vi "Autonomous Independent.vi"() -> ()   [LabVIEW 2017]
doc: "This VI is called when autonomous begins, and will automatically be terminated when autonomous ends. You can carry out timed or sensor driven robot movement independently without needing to return to the caller."
uses:
  <vilib>/Rock Robotics/WPI/DriverStation/WPI_DriverStationAllianceInfo.ctl
  <vilib>/Rock Robotics/WPI/Utilities/WPI_GetSetVariantRefNum.vi
  <vilib>/Rock Robotics/Network Tables/NT Read String.vi
  <vilib>/Rock Robotics/Network Tables/NT Write Numeric Array.vi
  <vilib>/Rock Robotics/WPI/RobotDrive/WPI_RobotDriveArcadeDrive_Standard(NoSaturation).vi
panel:
  in  "Test Recording":T1
  in  "Wrist Backward Delivery Recording":cluster{dbl, u32}[](array[cluster])
  in  "Shoulder Backward Delivery Recording":cluster{dbl, u32}[](array[cluster])
  in  "Wrist Delivery Recording":cluster{dbl, u32}[](array[cluster])
  in  "Shoulder Delivery Recording":cluster{dbl, u32}[](array[cluster])
  in  "Switch to Far Scale":T1
  in  "Switch to Close Scale":T1
  in  "Wrist Switch Delivery Recording":cluster{dbl, u32}[](array[cluster])
  in  "Start to Switch":T1
  out "Current Movement, for debugging":T2 {"Y Joystick Value" scale=1.0..-1.0; "X Joystick Value" scale=-1.0..1.0}
  in  "Array of robot movements":T3(array[cluster])=[{"X Joystick Value"=0.39393939393939403, "Y Joystick Value"=0.0, "Delay (sec)"=1.0, "Movement Name"="turn"}, {"X Joystick Value"=-0.3737373737373737, "Y Joystick Value"=0.0, "Delay (sec)"=1.0, "Movement Name"="turn back"}] {"Y Joystick Value" scale=1.0..-1.0; "X Joystick Value" scale=-1.0..1.0}
  # "Todo:\n-Invert the axis\n-Arm recordings\n-Floor Recordings\n-PID Values for Arms\n-PID Values for Floor"
  # "Be sure to right-click and choose Data Operations>>Make Current Value default if you want to save the array values with the VI"
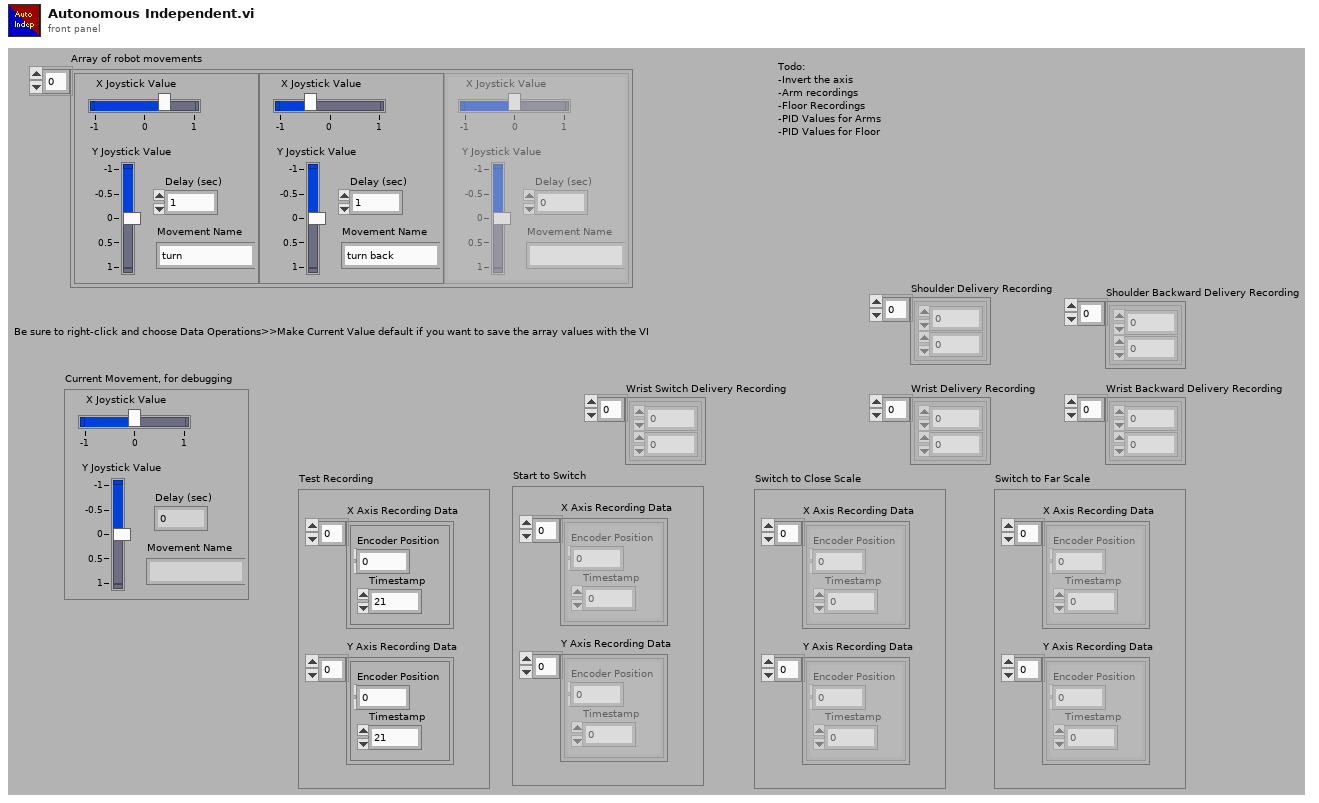
[diagram p1: front panel]
types:
  T1 = cluster{"X Axis Recording Data":cluster{"Encoder Position":dbl, "Timestamp":i32}[], "Y Axis Recording Data":cluster{"Encoder Position":dbl, "Timestamp":i32}[]}
  T2 = cluster{"X Joystick Value":dbl, "Y Joystick Value":dbl, "Delay (sec)":dbl, "Movement Name":string}
  T3 = cluster{"X Joystick Value":dbl, "Y Joystick Value":dbl, "Delay (sec)":dbl, "Movement Name":string}[]
  T4 = typedef "WPI_DriverStationAllianceInfo.ctl" = enum16{"Red", "Blue", "Invalid"}
  T5 = typedef "WPI_JoystickDevRef.ctl" = cluster{"Device":T6}
  T6 = typedef "WPI_JoystickDeviceEnum.ctl" = enum16{"USB 0", "USB 1", "USB 2", "USB 3", "USB 4", "USB 5"}
  T7 = typedef "WPI_RobotDriveDevRef.ctl" = cluster{"DevStatus":errorcluster, "Motors[]":T8[], "Square Inputs":bool, "Max Output":dbl}
  T8 = typedef "WPI_MotorControlDeviceRef.ctl" = cluster{"DeviceStatus":errorcluster, "Type":T9, "PWM":cluster{"PWM Channel":T10, "DeadBand":T11}, "CAN":cluster{"Device Number":u8, "SetOutput VI Ref":variant, "GetOutput VI Ref":variant, "Enable VI Ref":variant, "Disable VI Ref":variant, "Data":variant}, "Invert":bool, "DIO PWM":cluster{"PWM \"Enable\" Channel":T10, "DIOChannel":T12, "PWM Rate":dbl}}
  T9 = typedef "WPI_MotorControlType.ctl" = enum16{"PWM", "CAN", "DIO PWM"}
  T10 = typedef "FPGA_DIOPWMChannel.ctl" = enum8{"PWM 0", "PWM 1", "PWM 2", "PWM 3", "PWM 4", "PWM 5", "PWM 6", "PWM 7", "PWM 8", "PWM 9", "PWM MXP 0", "PWM MXP 1", "PWM MXP 2", "PWM MXP 3", "PWM MXP 4", "PWM MXP 5", "PWM MXP 6", "PWM MXP 7", "PWM MXP 8", "PWM MXP 9", "Invalid"}
  T11 = typedef "WPI_PWMDeadband.ctl" = cluster{"Name":string, "maxPositivePwm":i32, "minPositivePwm":i32, "centerPwm":i32, "maxNegativePwm":i32, "minNegativePwm":i32, "angularRange":u16}
  T12 = typedef "FPGA_DIOChannel.ctl" = enum8{"DIO 0", "DIO 1", "DIO 2", "DIO 3", "DIO 4", "DIO 5", "DIO 6", "DIO 7", "DIO 8", "DIO 9", "DIO MXP 0", "DIO MXP 1", "DIO MXP 2", "DIO MXP 3", "DIO MXP 4", "DIO MXP 5", "DIO MXP 6", "DIO MXP 7", "DIO MXP 8", "DIO MXP 9", "DIO MXP 10", "DIO MXP 11", "DIO MXP 12", "DIO MXP 13", "DIO MXP 14", "DIO MXP 15", "SPI Port CS1", "SPI Port CS2", "SPI Port CS3", "SPI Port MISO", "SPI Port MOSI", "Invalid"}
  T13 = typedef "WPI_EncoderDevRef.ctl" = cluster{"DevStatus":errorcluster, "EncoderIndex":T14, "CounterIndex":T15, "DistancePerCount":dbl, "Decoding Type":T16}
  T14 = typedef "FPGA_EncoderIdx.ctl" = enum8{"Enc 0", "Enc 1", "Enc 2", "Enc 3", "Enc 4", "Enc 5", "Enc 6", "Enc 7", "Invalid"}
  T15 = typedef "FPGA_CounterCtrSystemIndex.ctl" = enum8{"Ctr 0", "Ctr 1", "Ctr 2", "Ctr 3", "Ctr 4", "Ctr 5", "Ctr 6", "Ctr 7", "Invalid"}
  T16 = typedef "WPI_EncoderType.ctl" = enum16{"1x", "2x", "4x"}
  T17 = cluster{"refnum name":string, "EncoderDevRef":T13}
  T18 = cluster{"MotorControlDevRef":T8, "MotorControlDevRef":T8}
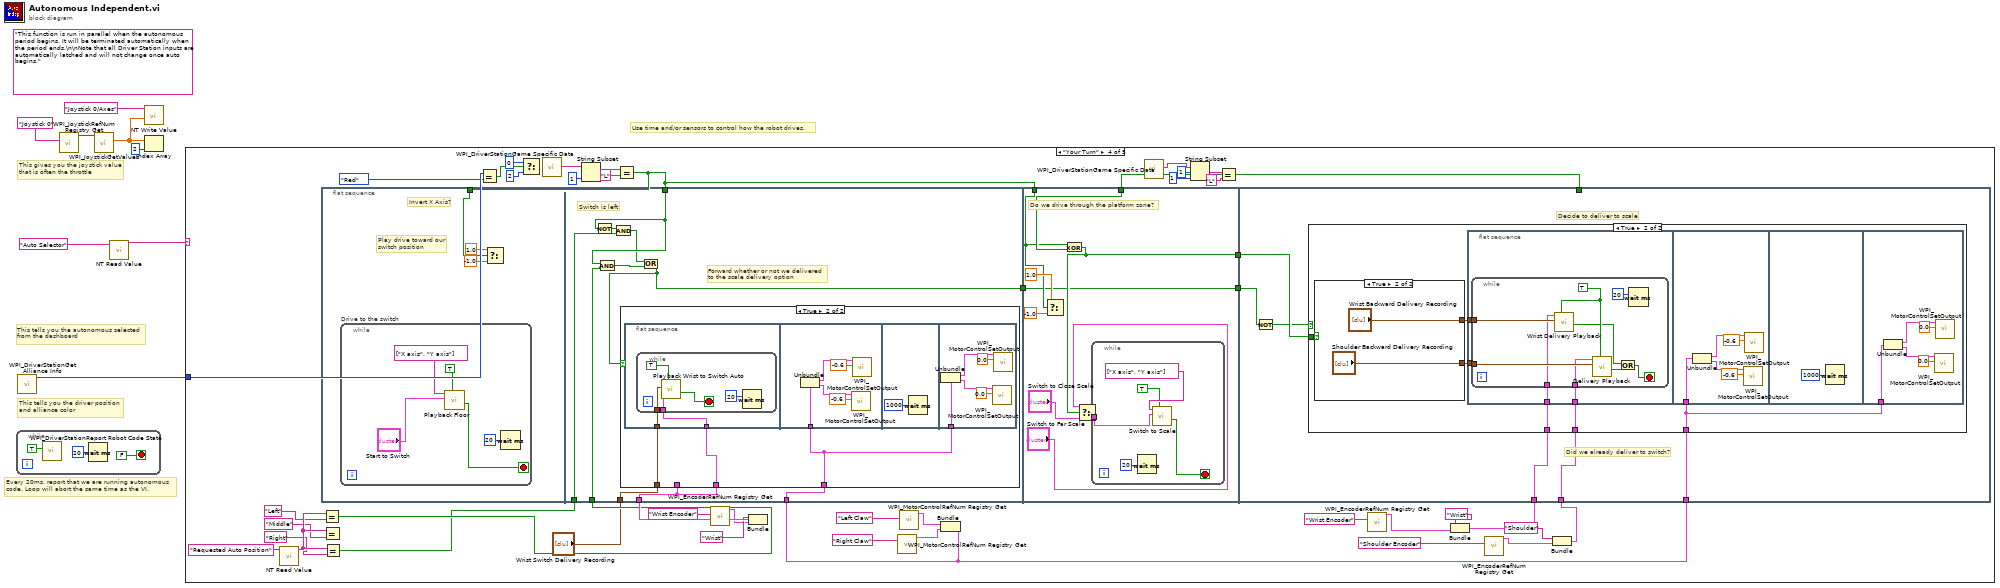
[diagram p0: block diagram]
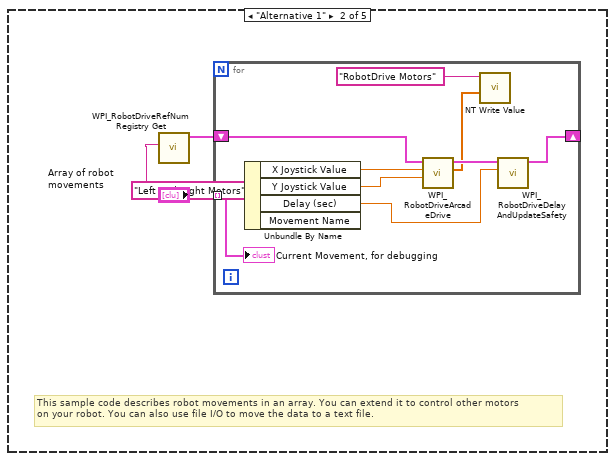
[diagram p3: hidden frame]
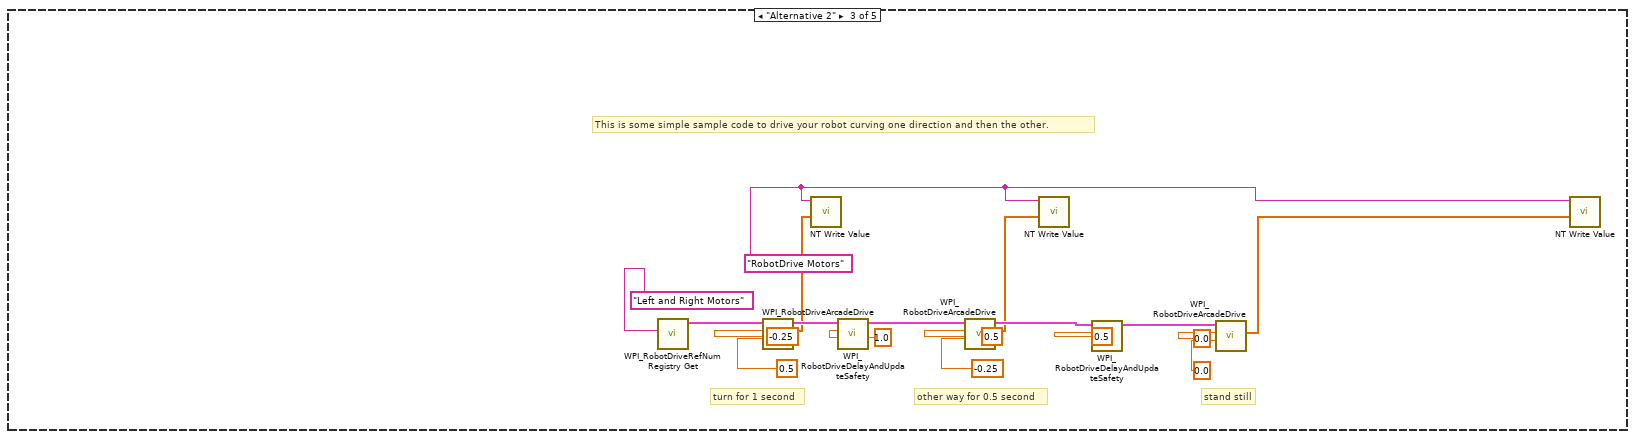
[diagram p4: hidden frame]
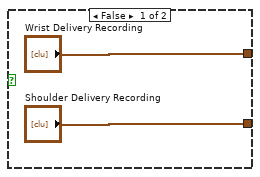
[diagram p7: hidden frame]
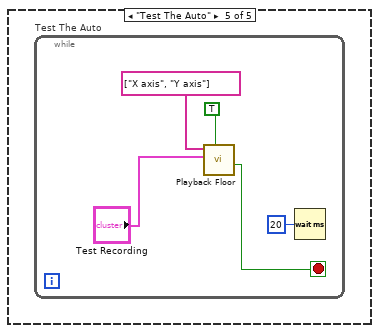
[diagram p8: hidden frame]
diagram:
  (unwired) "This function is run in parallel when the autonomous period begins. It will be terminated automatically when the period ends.\n\nNote that all Driver Station inputs are automatically latched and will not change once auto begins."
  # "This tells you the autonomous selected\nfrom the dashboard"
  # "Every 20ms, report that we are running autonomous\ncode. Loop will abort the same time as the VI."
  # "This gives you the joystick value\nthat is often the throttle"
  # "Use time and/or sensors to control how the robot drives."
  # "This tells you the driver position\nand alliance color"
  n1 = while {
    stop <- FALSE stop-if-true
    n2 = call <vilib>:"WPI_DriverStationReport Robot Code State.vi"("Autonomous"=TRUE) -> ()  [unwired: 10 in, 1 out]
    n3 = Wait (ms)(milliseconds to wait=u32 20) -> ()  [unwired: 1 out]
  }
  n4 = call <vilib>:"WPI_DriverStationGet Alliance Info.vi"() -> ("Alliance"=w1:T4)  [unwired: 11 out]
  n5 = call <vilib>:"WPI_JoystickRefNum Registry Get.vi"("refnum name"="Joystick 0") -> ("JoystickDevRef"=w7:T5)  [unwired: 1 in, 9 out]
  n6 = call <vilib>:"WPI_JoystickGetValues.vi"("JoystickDevRef"=w7) -> ("Axes"=w3:dbl[])  [unwired: 6 in, 4 out]
  n7 = call-poly <vilib>:"NT Read Value.vi"("Name"="Auto Selector") -> ("String"=w4:string)  [unwired: 9 in, 1 out]
  n8 = call-poly <vilib>:"NT Write Value.vi"("Numeric Array"=w3, "Name"="Joystick 0/Axes") -> ()  [unwired: 9 in, 1 out]
  n9 = Index Array(array=w3, index=2) -> ()  [unwired: 1 out]
  n10 = case shown="\"Your Turn\"" w4 {
    tunnel: w1 -> [_ _ _ w79 _]
    frame Default {
      # "You can put your main auto here, or you can right-click on the case and make any\nother frame be the default case."
      # "This is the frame that will execute if no selection is made, or if it is not recognized"
    }
    frame "Alternative 1" {
      # "This sample code describes robot movements in an array. You can extend it to control other motors\non your robot. You can also use file I/O to move the data to a text file."
      n11 = call <vilib>:"WPI_RobotDriveRefNum Registry Get.vi"("refnum name"="Left and Right Motors") -> ("RobotDriveDevRef"=w13:T7)  [unwired: 1 in, 9 out]
      n12 = for {
        shift-right: [w21] -> _
        shift-left: w13 -> [w22]
        tunnel: "Array of robot movements" -> [w17] mode=indexing
        n13 = Unbundle By Name(w17) -> ("X Joystick Value"=w20:dbl, "Y Joystick Value"=w19:dbl, "Delay (sec)"=w18:dbl)  [unwired: 1 out]
        n14 = call-poly <vilib>:"WPI_RobotDriveArcadeDrive.vi"("Y axis value"=w19, "X axis value"=w20, "RobotDriveDevRef"=w22) -> ("Motor Values"=w15:dbl[], "RobotDriveDevRef"=w23:T7)  [unwired: 1 in, 6 out]
        n15 = call-poly <vilib>:"NT Write Value.vi"("Numeric Array"=w15, "Name"="RobotDrive Motors") -> ()  [unwired: 9 in, 1 out]
        n16 = call <vilib>:"WPI_RobotDriveDelayAndUpdateSafety.vi"("Delay (s)"=w18, "RobotDriveDevRef"=w23) -> ("RobotDriveDevRef 2"=w21:T7)  [unwired: 8 in, 1 out]
        "Current Movement, for debugging" <- w17
      }
    }
    frame "Alternative 2" {
      w25 = "RobotDrive Motors" ("Name")
      # "This is some simple sample code to drive your robot curving one direction and then the other."
      # "stand still"
      # "other way for 0.5 second"
      # "turn for 1 second"
      n17 = call <vilib>:"WPI_RobotDriveRefNum Registry Get.vi"("refnum name"="Left and Right Motors") -> ("RobotDriveDevRef"=w41:T7)  [unwired: 1 in, 9 out]
      n18 = call-poly <vilib>:"WPI_RobotDriveArcadeDrive.vi"("Y axis value"=0.5 ("X axis value"), "X axis value"=-0.25, "RobotDriveDevRef"=w41) -> ("Motor Values"=w24:dbl[], "RobotDriveDevRef"=w34:T7)  [unwired: 1 in, 6 out]
      n19 = call-poly <vilib>:"NT Write Value.vi"("Numeric Array"=w24, "Name"=w25) -> ()  [unwired: 9 in, 1 out]
      n20 = call <vilib>:"WPI_RobotDriveDelayAndUpdateSafety.vi"("Delay (s)"=1.0, "RobotDriveDevRef"=w34) -> ("RobotDriveDevRef 2"=w35:T7)  [unwired: 8 in, 1 out]
      n21 = call-poly <vilib>:"WPI_RobotDriveArcadeDrive.vi"("Y axis value"=-0.25 ("X axis value"), "X axis value"=0.5, "RobotDriveDevRef"=w35) -> ("Motor Values"=w26:dbl[], "RobotDriveDevRef"=w36:T7)  [unwired: 1 in, 6 out]
      n22 = call-poly <vilib>:"NT Write Value.vi"("Numeric Array"=w26, "Name"=w25) -> ()  [unwired: 9 in, 1 out]
      n23 = call <vilib>:"WPI_RobotDriveDelayAndUpdateSafety.vi"("Delay (s)"=0.5, "RobotDriveDevRef"=w36) -> ("RobotDriveDevRef 2"=w37:T7)  [unwired: 8 in, 1 out]
      n24 = call-poly <vilib>:"WPI_RobotDriveArcadeDrive.vi"("Y axis value"=0.0 ("X axis value"), "X axis value"=0.0, "RobotDriveDevRef"=w37) -> ("Motor Values"=w27:dbl[])  [unwired: 1 in, 7 out]
      n25 = call-poly <vilib>:"NT Write Value.vi"("Numeric Array"=w27, "Name"=w25) -> ()  [unwired: 9 in, 1 out]
    }
    frame "Your Turn" {
      n26 = call-poly <vilib>:"NT Read Value.vi"("Name"="Requested Auto Position") -> ("String"=w70:string)  [unwired: 9 in, 1 out]
      n27 = flat-sequence {
        tunnel: w54 -> [w86]
        tunnel: w54 -> [w102]
        tunnel: w65 -> [w96]
        tunnel: w62 -> [w103]
        tunnel: w61 -> [w100]
        tunnel: w53 -> [w97]
        tunnel: "Wrist Switch Delivery Recording" -> [w95]
        tunnel: [w94] -> w42
        tunnel: w55 -> [w133]
        tunnel: w54 -> [w130]
        tunnel: [w126] -> w44
        tunnel: [w125] -> w43
        tunnel: w42 -> [w125]
        tunnel: w55 -> [_]
        tunnel: w53 -> [w144]
        tunnel: w50 -> [w143]
        tunnel: w45 -> [w142]
        tunnel: w44 -> [w141]
        tunnel: w43 -> [w139]
        frame #0 {
          # "Invert X Axis?"
          # "Play drive toward our\nswitch position"
          n28 = while "Drive to the switch" {
            stop <- w91 stop-if-true
            n29 = call "Playback Floor.vi"("Encoder Names"=string[] ["X axis", "Y axis"], "Floor Recording Data"="Start to Switch", "Playback"=TRUE) -> ("End of Playback"=w91:bool)  [unwired: 6 in, 1 out]
            n30 = Wait (ms)(milliseconds to wait=u32 20) -> ()  [unwired: 1 out]
          }
          n31 = Select(t=1.0, s=w86, f=-1.0) -> ()  [unwired: 1 out]
        }
        frame #1 {
          # "Forward whether or not we delivered\nto the scale delivery option"
          # "Switch is left"
          n32 = Not(x=w102) -> (.not. x?=w101:bool)
          n33 = And(x=w102, y=w103) -> (x .and. y?=w98:bool)
          n34 = And(x=w101, y=w100) -> (x .and. y?=w99:bool)
          n35 = Or(x=w99, y=w98) -> (x .or. y?=w94:bool)
          n36 = case shown="True" w94 {
            tunnel: w96 -> [_ _]
            tunnel: w97 -> [_ w106]
            tunnel: w96 -> [_ w105]
            tunnel: w95 -> [_ w104]
            frame False {
              # "Do nothing! We're not delivering here!"
            }
            frame True {
              n37 = flat-sequence {
                tunnel: w105 -> [w108]
                tunnel: w104 -> [w107]
                tunnel: w106 -> [w114]
                tunnel: w106 -> [w120]
                frame #0 {
                  n38 = while {
                    tunnel: w108 -> [w113]
                    tunnel: w107 -> [w110]
                    stop <- w112 stop-if-true
                    n39 = call "Playback Wrist to Switch Auto.vi"("Playback"=TRUE, "Encoder Recording Data"=w110, "Hardware In"=w113) -> ("Finished"=w112:bool)  [unwired: 7 in, 1 out]
                    n40 = Wait (ms)(milliseconds to wait=u32 20) -> ()  [unwired: 1 out]
                  }
                }
                frame #1 {
                  n41 = Unbundle(w114) -> ("MotorControlDevRef"=w118:T8, "MotorControlDevRef"=w117:T8)
                  n42 = call <vilib>:"WPI_MotorControlSetOutput.vi"("Output"=-0.6, "MotorControlDevRef"=w117) -> ()  [unwired: 7 in, 3 out]
                  n43 = call <vilib>:"WPI_MotorControlSetOutput.vi"("Output"=-0.6, "MotorControlDevRef"=w118) -> ()  [unwired: 7 in, 3 out]
                }
                frame #2 {
                  n44 = Wait (ms)(milliseconds to wait=u32 1000) -> ()  [unwired: 1 out]
                }
                frame #3 {
                  n45 = Unbundle(w120) -> ("MotorControlDevRef"=w124:T8, "MotorControlDevRef"=w123:T8)
                  n46 = call <vilib>:"WPI_MotorControlSetOutput.vi"("Output"=0.0, "MotorControlDevRef"=w123) -> ()  [unwired: 7 in, 3 out]
                  n47 = call <vilib>:"WPI_MotorControlSetOutput.vi"("Output"=0.0, "MotorControlDevRef"=w124) -> ()  [unwired: 7 in, 3 out]
                }
              }
            }
          }
        }
        frame #2 {
          # "Do we drive through the platform zone?"
          n48 = Select(t=1.0, s=w130, f=-1.0) -> ()  [unwired: 1 out]
          n49 = Exclusive Or(1:w133, 2:w130) -> (0:w126:bool)
          n50 = Select(t="Switch to Far Scale", s=w126, f="Switch to Close Scale") -> (s? t:f=w127:T1)
          n51 = while {
            tunnel: w127 -> [w134]
            stop <- w137 stop-if-true
            n52 = Wait (ms)(milliseconds to wait=u32 20) -> ()  [unwired: 1 out]
            n53 = call "Switch to Scale.vi"("Encoder Names"=string[] ["X axis", "Y axis"], "Floor Recording Data"=w134, "Playback"=TRUE) -> ("End of Playback"=w137:bool)  [unwired: 6 in, 1 out]
          }
        }
        frame #3 {
          # "Did we already deliver to switch?"
          # "Decide to deliver to scale"
          n54 = Not(x=w139) -> (.not. x?=w140:bool)
          n55 = case shown="True" w140 {
            tunnel: w144 -> [_ w150]
            tunnel: w143 -> [_ w147]
            tunnel: w142 -> [_ w146]
            tunnel: w141 -> [_ w145]
            frame False {
              # "We shall deliver nothing! ah ah ah..."
            }
            frame True {
              n56 = case shown="True" w145 {
                tunnel: ["Shoulder Delivery Recording" "Shoulder Backward Delivery Recording"] -> w149
                tunnel: ["Wrist Delivery Recording" "Wrist Backward Delivery Recording"] -> w148
                frame False {
                }
                frame True {
                }
              }
              n57 = flat-sequence {
                tunnel: w149 -> [w158]
                tunnel: w148 -> [w157]
                tunnel: w147 -> [w156]
                tunnel: w146 -> [w155]
                tunnel: w150 -> [w168]
                tunnel: w150 -> [w174]
                frame #0 {
                  n58 = while {
                    tunnel: w158 -> [w166]
                    tunnel: w157 -> [w165]
                    tunnel: w156 -> [w163]
                    tunnel: w155 -> [w162]
                    stop <- w159 stop-if-true
                    w164 = TRUE
                    n59 = call "Wrist Delivery Playback.vi"("Playback"=w164, "Encoder Recording Data"=w165, "Hardware In"=w162) -> ("Playback Finished"=w160:bool)  [unwired: 7 in, 1 out]
                    n60 = call "Delivery Playback.vi"("Playback"=w164, "Encoder Recording Data"=w166, "Hardware In"=w163) -> ("Finish Playback"=w161:bool)  [unwired: 7 in, 1 out]
                    n61 = Or(x=w160, y=w161) -> (x .or. y?=w159:bool)
                    n62 = Wait (ms)(milliseconds to wait=u32 20) -> ()  [unwired: 1 out]
                  }
                }
                frame #1 {
                  n63 = Unbundle(w168) -> ("MotorControlDevRef"=w172:T8, "MotorControlDevRef"=w171:T8)
                  n64 = call <vilib>:"WPI_MotorControlSetOutput.vi"("Output"=-0.6, "MotorControlDevRef"=w171) -> ()  [unwired: 7 in, 3 out]
                  n65 = call <vilib>:"WPI_MotorControlSetOutput.vi"("Output"=-0.6, "MotorControlDevRef"=w172) -> ()  [unwired: 7 in, 3 out]
                }
                frame #2 {
                  n66 = Wait (ms)(milliseconds to wait=u32 1000) -> ()  [unwired: 1 out]
                }
                frame #3 {
                  n67 = Unbundle(w174) -> ("MotorControlDevRef"=w178:T8, "MotorControlDevRef"=w177:T8)
                  n68 = call <vilib>:"WPI_MotorControlSetOutput.vi"("Output"=0.0, "MotorControlDevRef"=w177) -> ()  [unwired: 7 in, 3 out]
                  n69 = call <vilib>:"WPI_MotorControlSetOutput.vi"("Output"=0.0, "MotorControlDevRef"=w178) -> ()  [unwired: 7 in, 3 out]
                }
              }
            }
          }
        }
      }
      n70 = Equal?(x=w70, y="Left") -> (x = y?=w62:bool)
      n71 = Equal?(x=w70, y="Middle") -> ()  [unwired: 1 out]
      n72 = Equal?(x=w70, y="Right") -> (x = y?=w61:bool)
      n73 = Equal?(x=w79, y=WPI_DriverStationAllianceInfo."Red") -> (x = y?=w77:bool)
      n74 = Select(t=0 ("length (rest)"), s=w77, f=2 ("length (rest)")) -> ()  [unwired: 1 out]
      n75 = call <vilib>:"WPI_DriverStationGame Specific Data.vi"() -> ("Game Specific Data"=w85:string)  [unwired: 11 in]
      n76 = String Subset(string=w85, length (rest)=1 ("length (rest)")) -> (substring=w83:string)  [unwired: 1 in]
      n77 = Equal?(x=w83, y="L") -> (x = y?=w54:bool)
      n78 = call <vilib>:"WPI_EncoderRefNum Registry Get.vi"("refnum name"="Wrist Encoder") -> ("EncoderDevRef"=w63:T13)  [unwired: 9 in, 1 out]
      n79 = Bundle("refnum name"="Wrist", "EncoderDevRef"=w63) -> (w65:T17)  [unwired: 1 in]
      n80 = call <vilib>:"WPI_MotorControlRefNum Registry Get.vi"("refnum name"="Right Claw") -> ("MotorControlDevRef"=w59:T8)  [unwired: 9 in, 1 out]
      n81 = call <vilib>:"WPI_MotorControlRefNum Registry Get.vi"("refnum name"="Left Claw") -> ("MotorControlDevRef"=w60:T8)  [unwired: 9 in, 1 out]
      n82 = Bundle("MotorControlDevRef"=w60, "MotorControlDevRef"=w59) -> (w53:T18)  [unwired: 1 in]
      n83 = call <vilib>:"WPI_DriverStationGame Specific Data.vi"() -> ("Game Specific Data"=w75:string)  [unwired: 11 in]
      n84 = String Subset(string=w75, offset (0)=1, length (rest)=1 ("length (rest)")) -> (substring=w73:string)
      n85 = Equal?(x=w73, y="L") -> (x = y?=w55:bool)
      n86 = call <vilib>:"WPI_EncoderRefNum Registry Get.vi"("refnum name"="Wrist Encoder") -> ("EncoderDevRef"=w47:T13)  [unwired: 9 in, 1 out]
      n87 = Bundle("Wrist", "EncoderDevRef"=w47) -> (w45:cluster{string, "EncoderDevRef":T13})  [unwired: 1 in]
      n88 = call <vilib>:"WPI_EncoderRefNum Registry Get.vi"("refnum name"="Shoulder Encoder") -> ("EncoderDevRef"=w48:T13)  [unwired: 9 in, 1 out]
      n89 = Bundle("Shoulder", "EncoderDevRef"=w48) -> (w50:cluster{string, "EncoderDevRef":T13})  [unwired: 1 in]
    }
    frame "Test The Auto" {
      n90 = while "Test The Auto" {
        stop <- w181 stop-if-true
        n91 = call "Playback Floor.vi"("Encoder Names"=string[] ["X axis", "Y axis"], "Floor Recording Data"="Test Recording", "Playback"=TRUE) -> ("End of Playback"=w181:bool)  [unwired: 6 in, 1 out]
        n92 = Wait (ms)(milliseconds to wait=u32 20) -> ()  [unwired: 1 out]
      }
    }
  }
